vi "WritePointToCurGraph.vi"(9 "PointArray":cluster{"X":dbl, "Y":dbl}[](array[cluster])=[{"X"=1.0, "Y"=2.0}, {"X"=3.0, "Y"=4.0}], 10 "游标标识":enum16{"Cursor 01", "Cursor 02"}(ring), 11 "PicIn":picture) -> (3 "PicOut":picture)   [LabVIEW 2012, in "WaveGraphX.xctl"]
uses:
  WaveGraphX.xctl
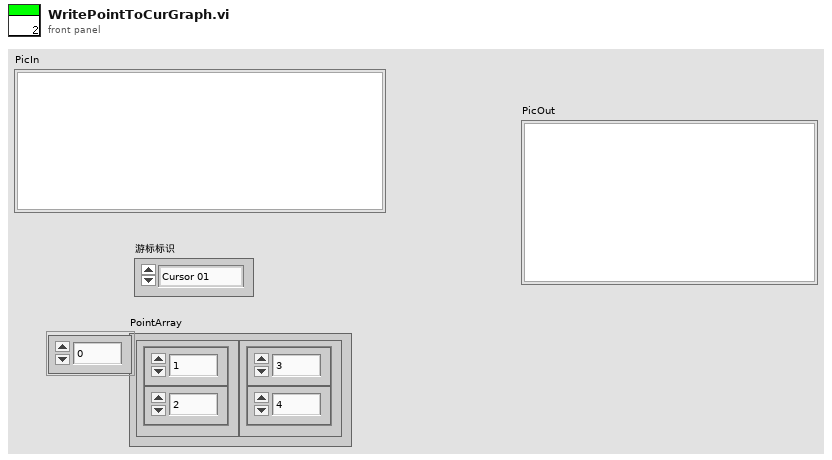
[diagram p1: front panel]
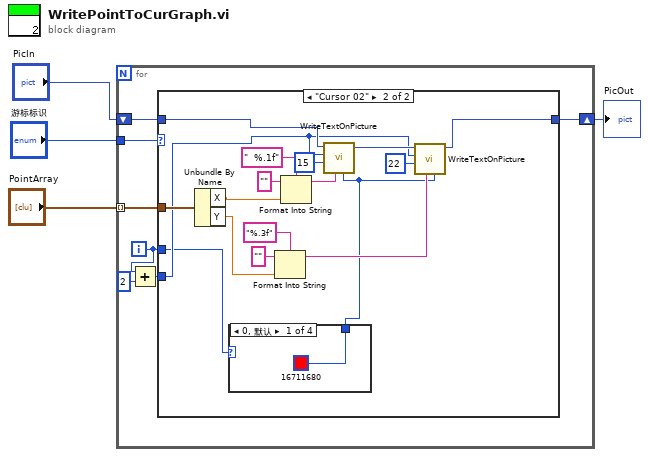
[diagram p0: block diagram]
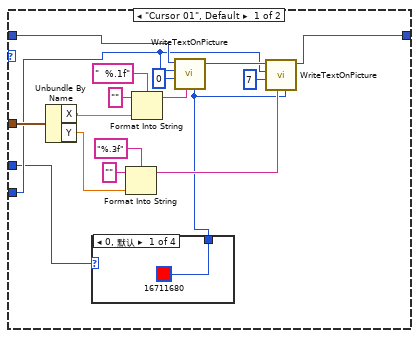
[diagram p2: hidden frame]
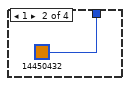
[diagram p3: hidden frame]
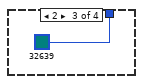
[diagram p4: hidden frame]
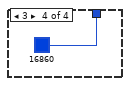
[diagram p5: hidden frame]
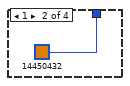
[diagram p6: hidden frame]
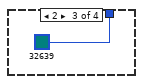
[diagram p7: hidden frame]
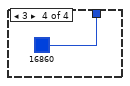
[diagram p8: hidden frame]
diagram:
  n1 = for {
    tunnel: "PointArray" -> [w10] mode=indexing
    tunnel: "游标标识" -> [w11]
    shift-right: [w6] -> w1
    shift-left: "PicIn" -> [w9]
    i -> [w5]
    n2 = Add(x=w5, y=2) -> (x+y=w7:i32)
    n3 = case shown="\"Cursor 02\"" w11 {
      tunnel: w10 -> [w28 w49]
      tunnel: w9 -> [w21 w42]
      tunnel: w7 -> [w17 w38]
      tunnel: [w14 w35] -> w6
      tunnel: w5 -> [w13 w34]
      frame "Cursor 01", Default {
        n4 = Unbundle By Name(w28) -> ("X"=w22:dbl, "Y"=w25:dbl)
        n5 = case shown="0, 默认" w13 {
          tunnel: [u32 16711680 ("plot color") u32 14450432 ("plot color 2") u32 32639 ("plot color 3") u32 16860 ("plot color 4")] -> w12
          frame 0, Default {
          }
          frame 1 {
          }
          frame 2 {
          }
          frame 3 {
          }
        }
        n6 = Format Into String(format string="%.3f" ("格式字符串"), initial string="" ("初始字符串"), w25) -> (resulting string=w15:string)  [unwired: 1 in, 1 out]
        n7 = Format Into String(format string="  %.1f" ("格式字符串"), initial string="" ("初始字符串"), w22) -> (resulting string=w20:string)  [unwired: 1 in, 1 out]
        n8 = call "WriteTextOnPicture.vi"("颜色"=w12, "文本"=w20, "列索引"=u32 0, "行索引"=w17, "Origin Picture"=w21) -> ("Picture Out"=w18:picture)  [unwired: 6 in]
        n9 = call "WriteTextOnPicture.vi"("颜色"=w12, "文本"=w15, "列索引"=u32 7, "行索引"=w17, "Origin Picture"=w18) -> ("Picture Out"=w14:picture)  [unwired: 6 in]
      }
      frame "Cursor 02" {
        n10 = Unbundle By Name(w49) -> ("X"=w43:dbl, "Y"=w46:dbl)
        n11 = case shown="0, 默认" w34 {
          tunnel: [u32 16711680 ("plot color") u32 14450432 ("plot color 2") u32 32639 ("plot color 3") u32 16860 ("plot color 4")] -> w33
          frame 0, Default {
          }
          frame 1 {
          }
          frame 2 {
          }
          frame 3 {
          }
        }
        n12 = Format Into String(format string="%.3f" ("格式字符串"), initial string="" ("初始字符串"), w46) -> (resulting string=w36:string)  [unwired: 1 in, 1 out]
        n13 = Format Into String(format string="  %.1f" ("格式字符串"), initial string="" ("初始字符串"), w43) -> (resulting string=w41:string)  [unwired: 1 in, 1 out]
        n14 = call "WriteTextOnPicture.vi"("颜色"=w33, "文本"=w41, "列索引"=u32 15, "行索引"=w38, "Origin Picture"=w42) -> ("Picture Out"=w39:picture)  [unwired: 6 in]
        n15 = call "WriteTextOnPicture.vi"("颜色"=w33, "文本"=w36, "列索引"=u32 22, "行索引"=w38, "Origin Picture"=w39) -> ("Picture Out"=w35:picture)  [unwired: 6 in]
      }
    }
  }
  "PicOut" <- w1
